vi "example2.vi"() -> ()   [LabVIEW 2010]
uses:
  User32dllAPI.SetWindowPos.Flag.ctl
panel:
  out "error out":errorcluster
  in  "WinPos":cluster{"X":i32, "Y":i32, "dX":i32, "dY":i32}={"X"=100, "Y"=100, "dX"=200, "dY"=500}
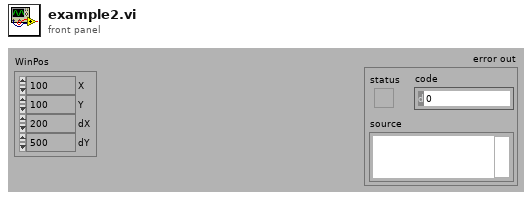
[diagram p1: front panel]
types:
  T1 = typedef "User32dllAPI.SetWindowPos.Flag.ctl" = u32
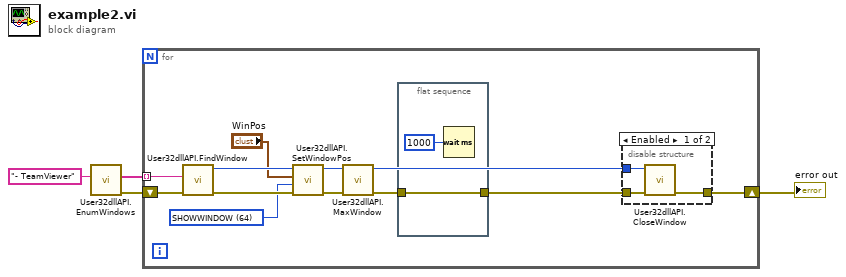
[diagram p0: block diagram]
diagram:
  n1 = call "User32dllAPI.EnumWindows.vi"("Pattern"="- TeamViewer") -> ("error out"=w3:errorcluster, "WindowName"=w2:string[])  [unwired: 7 in, 2 out]
  n2 = for {
    tunnel: w2 -> [w11] mode=indexing
    shift-right: [w10] -> w4
    shift-left: w3 -> [w12]
    w13 = T1 64 items=["NOSIZE"=1, "NOMOVE"=2, "NOZORDER"=4, "NOREDRAW"=8, "NOACTIVATE"=16, "DRAWFRAME"=32, "SHOWWINDOW"=64, "HIDEWINDOW"=128, "NOCOPYBITS"=256, "NOSENDCHANGING"=1024, "DEFERERASE"=8192, "ASYNCWINDOWPOS"=16384] ("User32dllAPI.SetWindowPos.Flag")
    n3 = call "User32dllAPI.FindWindow.vi"("error in (no error)"=w12, "WindowName"=w11) -> ("error out"=w16:errorcluster, "hWnd"=w15:i32)  [unwired: 8 in]
    n4 = call "User32dllAPI.SetWindowPos.vi"("error in (no error)"=w16, "Flags (SHOWWINDOW)"=w13, "WinPos"="WinPos", "hWnd in"=w15) -> ("error out"=w9:errorcluster, "hWnd out"=w8:i32)  [unwired: 6 in]
    n5 = call "User32dllAPI.MaxWindow.vi"("error in (no error)"=w9, "hWnd"=w8) -> ("error out"=w7:errorcluster, "hWnd out"=w5:i32)  [unwired: 8 in]
    n6 = flat-sequence {
      tunnel: [w21] -> w6
      tunnel: w7 -> [w21]
      frame #0 {
        n7 = Wait (ms)(milliseconds to wait=u32 1000) -> ()  [unwired: 1 out]
      }
    }
    n8 = disable-structure shown="Enabled" {
      disable-tunnel: [w19 w20] -> w10
      disable-tunnel: w6 -> [w18 w20]
      disable-tunnel: w5 -> [w17 _]
      frame Enabled {
        n9 = call "User32dllAPI.CloseWindow.vi"("error in (no error)"=w18, "hWnd"=w17) -> ("error out"=w19:errorcluster)  [unwired: 8 in, 1 out]
      }
      frame Disabled {
      }
    }
  }
  "error out" <- w4
